vi "Make shift signal-old.vi"(6 "postcycles":dbl, 7 "Output freq (Hz)":dbl=50.0, 8 "sinamp":dbl=20.0 caption="sineamp", 9 "sinfreq":dbl=1.5 caption="sinefreq", 10 "total time":dbl=20.0, 11 "pulse data":T1) -> (3 "sine signal":dbl[](array[numeric]))   [LabVIEW 2013]
uses:
  Pulse data.ctl
  <vilib>/Analysis/1siggen.llb/Ramp Pattern by Samples.vi
  <vilib>/Analysis/1siggen.llb/Ramp Pattern by Delta.vi
  <vilib>/Analysis/NI_AALBase.lvlib
  <vilib>/gmath/NI_Gmath.lvlib
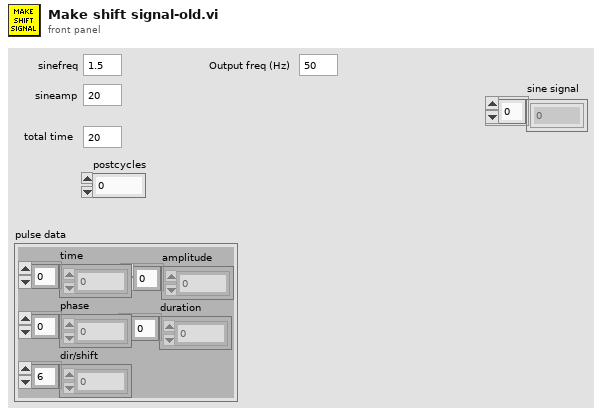
[diagram p1: front panel]
types:
  T1 = typedef "Pulse data.ctl" = cluster{"time":dbl[], "phase":dbl[], "dir/shift":dbl[], "amplitude":dbl[], "duration":dbl[]}
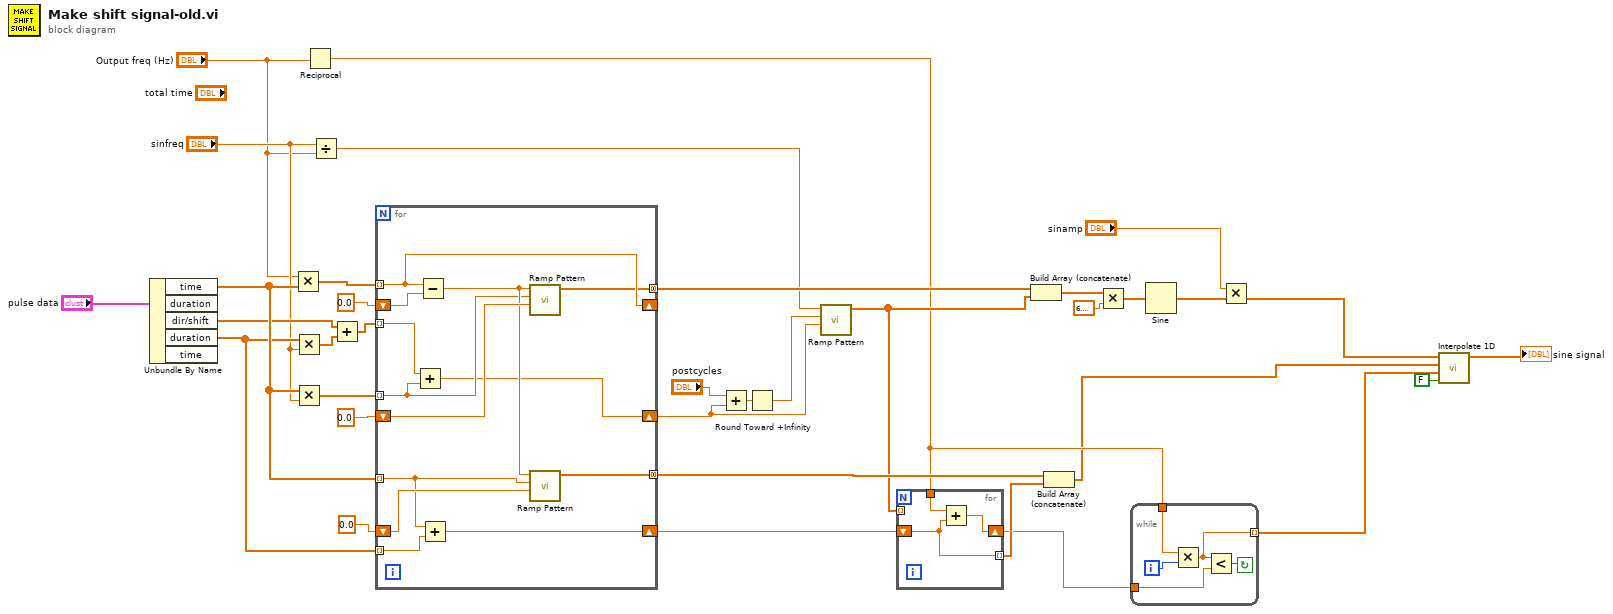
[diagram p0: block diagram]
diagram:
  n1 = Unbundle By Name("pulse data") -> ("time"=w32:dbl[], "dir/shift"=w26:dbl[], "duration"=w24:dbl[])  [unwired: 2 out]
  n2 = Multiply(x="Output freq (Hz)", y=w32) -> (x*y=w33:dbl[])
  n3 = Multiply(x=w24, y="sinfreq") -> (x*y=w27:dbl[])
  n4 = Multiply(x=w32, y="sinfreq") -> (x*y=w30:dbl[])
  n5 = Reciprocal(x="Output freq (Hz)") -> (1/x=w8:dbl)
  n6 = Divide(x="sinfreq", y="Output freq (Hz)") -> (x/y=w17:dbl)
  n7 = Add(x=w26, y=w27) -> (x+y=w28:dbl[])
  n8 = for {
    tunnel: w33 -> [w38] mode=indexing
    shift-right: [w38] -> _
    shift-left: 0.0 -> [w48]
    tunnel: w32 -> [w43] mode=indexing
    shift-right: [w42] -> w14
    shift-left: 0.0 -> [w45]
    tunnel: w30 -> [w41] mode=indexing
    shift-right: [w39] -> w23
    shift-left: 0.0 -> [w47]
    tunnel: w24 -> [w44] mode=indexing
    tunnel: w28 -> [w40] mode=indexing
    tunnel: [w37] -> w25 mode=concatenating
    tunnel: [w36] -> w20 mode=concatenating
    n9 = Add(x=w40, y=w41) -> (x+y=w39:dbl)
    n10 = Subtract(x=w38, y=w48) -> (x-y=w46:dbl)
    n11 = Add(x=w43, y=w44) -> (x+y=w42:dbl)
    n12 = call-poly <vilib>:"Ramp Pattern.vi"("start"=w47, "end"=w41, "samples"=w46) -> ("Ramp Pattern"=w37:dbl[])  [unwired: 7 in, 1 out]
    n13 = call-poly <vilib>:"Ramp Pattern.vi"("start"=w45, "end"=w43, "samples"=w46) -> ("Ramp Pattern"=w36:dbl[])  [unwired: 7 in, 1 out]
  }
  n14 = Add(x="postcycles", y=w23) -> (x+y=w22:dbl)
  n15 = Round Toward +Infinity(x=w22) -> (ceil(x): smallest int >= x=w21:dbl)
  n16 = call-poly <vilib>:"Ramp Pattern.vi"("start"=w23, "end"=w21, "delta"=w17) -> ("Ramp Pattern"=w16:dbl[])  [unwired: 6 in, 2 out]
  n17 = for {
    tunnel: w16 -> [_] mode=indexing
    shift-right: [w51] -> w9
    shift-left: w14 -> [w49]
    tunnel: w8 -> [w50]
    tunnel: [w49] -> w13 mode=indexing
    n18 = Add(x=w50, y=w49) -> (x+y=w51:dbl)
  }
  n19 = Build Array (concatenate)(w25, w16) -> (w12:dbl[])
  n20 = Build Array (concatenate)(w20, w13) -> (w6:dbl[])
  n21 = Multiply(x=w12, y=6.283185307179586) -> (x*y=w10:dbl[])
  n22 = while {
    tunnel: w9 -> [w54]
    tunnel: w8 -> [w55]
    tunnel: [w52] -> w5 mode=indexing
    i -> [w56]
    stop <- w53 continue-if-true
    n23 = Multiply(x=w55, y=w56) -> (x*y=w52:dbl)
    n24 = Less?(x=w52, y=w54) -> (x < y?=w53:bool)
  }
  n25 = Sine(x=w10) -> (sin(x)=w7:dbl[])
  n26 = Multiply(x="sinamp", y=w7) -> (x*y=w2:dbl[])
  n27 = call <vilib>:"Interpolate 1D.vi"("X is monotonic"=FALSE, "xi"=w5, "X"=w6, "Y"=w2) -> ("yi"=→"sine signal":dbl[])  [unwired: 5 in, 2 out]
